vi "Unregister.vi"(11 "client handle":T1) -> ()   [LabVIEW 2012]
uses:
  <vilib>/httpClient/ClientHandle.ctl
  <vilib>/httpClient/LabVIEWHTTPClient.lvlib
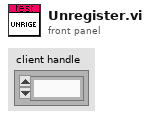
[diagram p1: front panel]
types:
  T1 = typedef "LabVIEWHTTPClient.lvlib/ClientHandle.ctl" = refnum<k1>
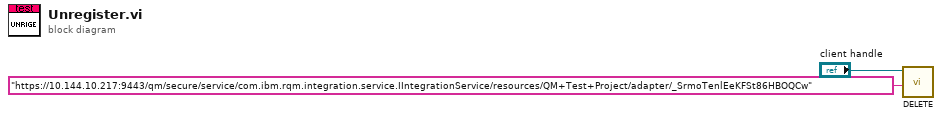
[diagram p0: block diagram]
diagram:
  n1 = call <vilib>:"DELETE.vi"("client handle"="client handle", "url"="https://10.144.10.217:9443/qm/secure/service/com.ibm.rqm.integration.service.IIntegrationService/resources/QM+Test+Project/adapter/_SrmoTenlEeKFSt86HBOQCw") -> ()  [unwired: 10 in, 4 out]
